vi "Set Counter Settings.vi"(8 "error in":errorcluster, 10 "Counter Settings":T1={"Counter Setpoint Mode"=enum."No setpoint change (default)", "Counter Limit"=0.0, "Unit"="ls", "Counter Mode"=enum."Counter off (default)", "Counter New Setpoint"=0}, 11 "Device":T4) -> (0 "error out":errorcluster)   [LabVIEW 2024, in "FlexiFlowInterfaceCH2.lvlib"]
doc: "Set the counter settings.\n_____\nCreated using DQMH Event Scripter 7.0.1.1316."
uses:
  FlexiFlowInterfaceCH2.lvlib
  FlexiFlowDevice--enum.ctl
  Counter Settings--cluster.ctl
  Modbus Flexi-Flow API/Counter Setpoint Mode--enum.ctl
  Modbus Flexi-Flow API/Counter Modes--enum.ctl
  Set Counter Settings Argument--cluster.ctl
  Modbus Flexi-Flow API/Bronkhorst Flexi-Flow ModbusTCP API.lvlib
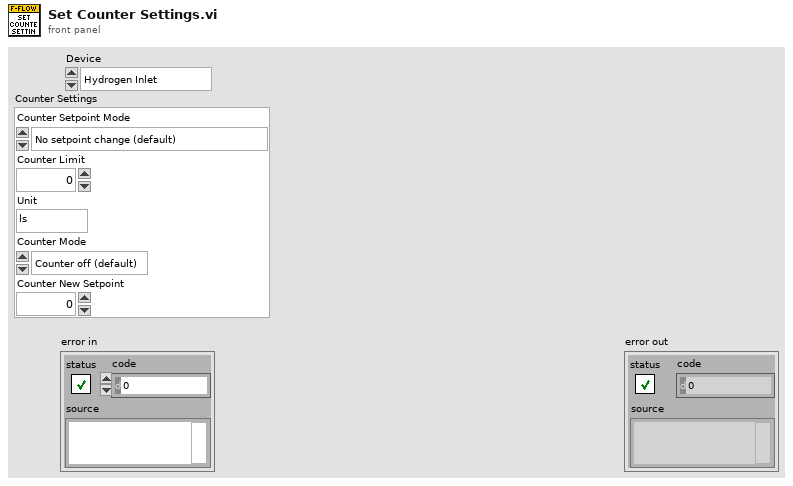
[diagram p1: front panel]
types:
  T1 = typedef "FlexiFlowInterfaceCH2.lvlib/Counter Settings--cluster.ctl" = cluster{"Counter Setpoint Mode":T2, "Counter Limit":sgl, "Unit":string, "Counter Mode":T3, "Counter New Setpoint":u16}
  T2 = typedef "Bronkhorst Flexi-Flow ModbusTCP API.lvlib/Counter Setpoint Mode--enum.ctl" = enum16{"No setpoint change (default)", "Change setpoint to Counter new setpoint"}
  T3 = typedef "Bronkhorst Flexi-Flow ModbusTCP API.lvlib/Counter Modes--enum.ctl" = enum16{"Counter off (default)", "Counting up continuously", "Counting up until limit reached"}
  T4 = typedef "FlexiFlowInterfaceCH2.lvlib/FlexiFlowDevice--enum.ctl" = enum16{"Hydrogen Inlet", "Nitrogen Inlet", "Cathode Outlet", "Anode Outlet"}
  T5 = typedef "FlexiFlowInterfaceCH2.lvlib/Set Counter Settings Argument--cluster.ctl" = cluster{"Device":T4, "Counter Settings":T1}
  T6 = typedef "FlexiFlowInterfaceCH2.lvlib/Request Events--cluster.ctl" = cluster{"Stop Module":refnum<user-event>, "Show Panel":refnum<user-event>, "Hide Panel":refnum<user-event>, "Get Module Execution Status":refnum<user-event>, "Show Diagram":refnum<user-event>, "Change Panel":refnum<user-event>, "Private":cluster{"Start Modbus Polling Helper Loop":refnum<user-event>, "Sleep Modbus Polling Helper Loop":refnum<user-event>, "Wake Connection Helper Loop":refnum<user-event>, "Sleep Connection Helper Loop":refnum<user-event>}, "Initialise Modbus Connections":refnum<user-event>, "Read Fmeasure":refnum<user-event>, "Set Modbus Configuration":refnum<user-event>, "Wink Devices":refnum<user-event>, "Read All FlexiFlow Device States":refnum<user-event>, "Wink Device":refnum<user-event>, "Set Control Function":refnum<user-event>, "Set Flow Setpoint":refnum<user-event>, "Set Backpressure Setpoint":refnum<user-event>, "Set Forward Pressure SP":refnum<user-event>, "Set Capacity Unit":refnum<user-event>, "Set Flow Capacity Unit":refnum<user-event>, "Set Setpoint Slope":refnum<user-event>, "Set Counter Settings":refnum<user-event>, "Reset All Device Counters":refnum<user-event>, "Read Device User Tag":refnum<user-event>, "Set Device User Tag":refnum<user-event>, "Read Counter Unit":refnum<user-event>, "Set Control Mode":refnum<user-event>, "Get Device Configuration":refnum<user-event>}
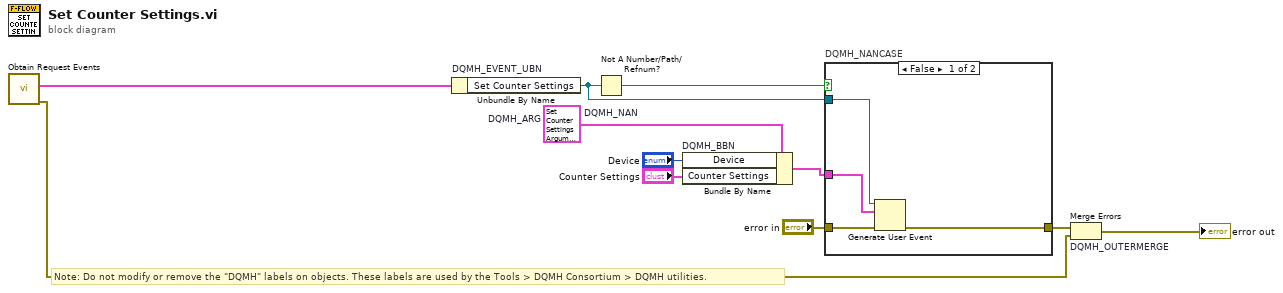
[diagram p0: block diagram]
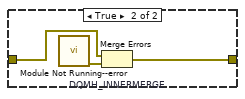
[diagram p2: hidden frame]
diagram:
  w5 = T5 {"Device"=enum."Hydrogen Inlet", "Counter Settings"={"Counter Setpoint Mode"=enum."No setpoint change (default)", "Counter Limit"=0.0, "Unit"="ls", "Counter Mode"=enum."Counter off (default)", "Counter New Setpoint"=0}}  # DQMH_ARG
  # "Note: Do not modify or remove the \"DQMH\" labels on objects. These labels are used by the Tools > DQMH Consortium > DQMH utilities."
  n1 = call "Obtain Request Events.vi"() -> ("error out"=w4:errorcluster, "FlexiFlowInterfaceCH2 Request Events"=w3:T6)  [unwired: 10 in]
  n2 = Unbundle By Name "DQMH_EVENT_UBN"(w3) -> ("Set Counter Settings"=w7:refnum<user-event>)
  n3 = Not A Number/Path/Refnum? "DQMH_NAN"(number/path/refnum=w7) -> (NaN/Path/Refnum?=w8:bool)
  n4 = Bundle By Name "DQMH_BBN"(cluster=w5, "Device"="Device", "Counter Settings"="Counter Settings") -> (w9:T5)
  n5 = case "DQMH_NANCASE" shown="False" w8 {
    tunnel: "error in" -> [w15 w18]
    tunnel: [w14 w17] -> w6
    tunnel: w7 -> [w13 _]
    tunnel: w9 -> [w12 _]
    frame False {
      n6 = Generate User Event(user event=w13, event data cluster=w12, error in=w15) -> (error out=w14:errorcluster)  [unwired: 1 in, 1 out]
    }
    frame True {
      n7 = call "Module Not Running--error.vi"() -> ("error out"=w16:errorcluster)  [unwired: 11 in]
      n8 = Merge Errors "DQMH_INNERMERGE"(w18, w16) -> (w17:errorcluster)
    }
  }
  n9 = Merge Errors "DQMH_OUTERMERGE"(w6, w4) -> (→"error out":errorcluster)
